vi "Smooth Move Window.vi"(8 "error in (no error)":errorcluster, 10 "Front Panel Window:Window Bounds":T1, 11 "VI in":refnum<vi>) -> (0 "error out":errorcluster, 3 "VI out":refnum<vi>)   [LabVIEW 2012, in "Win8uiDemo.lvlib" / "Flyout.lvclass"]
uses:
  Flyout.lvclass
  <vilib>/Utility/miscctls.llb/LVRectTypeDef.ctl
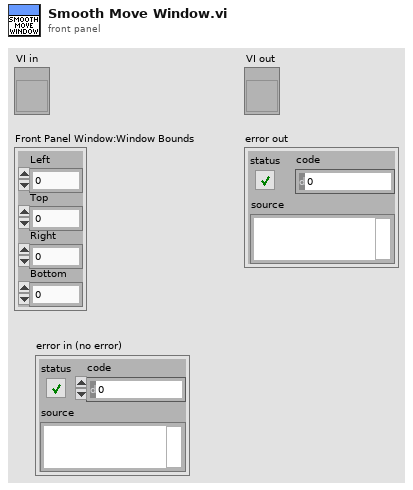
[diagram p1: front panel]
types:
  T1 = typedef "LVRectTypeDef.ctl" = cluster{"Left":i16, "Top":i16, "Right":i16, "Bottom":i16}
  T2 = cluster{"Left":dbl, "Top":dbl, "Right":dbl, "Bottom":dbl}
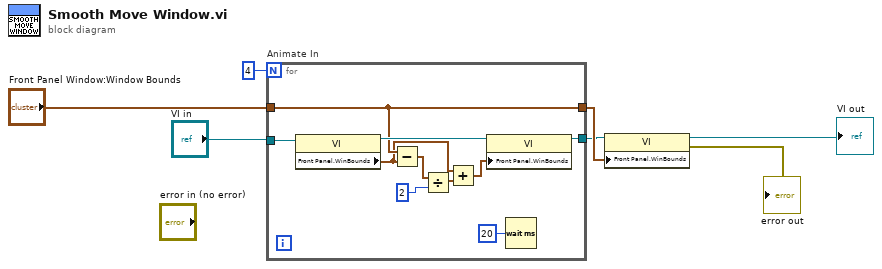
[diagram p0: block diagram]
diagram:
  n1 = for "Animate In" {
    N: 4 -> [_]
    tunnel: "VI in" -> [w17]
    tunnel: "Front Panel Window:Window Bounds" -> [w11]
    tunnel: [w12] -> w6
    tunnel: [w11] -> w7
    n2 = property class="VI"(reference=w17) -> (reference out=w13:refnum<vi>, "Front Panel.WinBounds"=w9:T1)  [unwired: 1 in, 1 out]
    n3 = Subtract(x=w11, y=w9) -> (x-y=w15:T1)
    n4 = Divide(x=w15, y=i16 2) -> (x/y=w10:T2)
    n5 = Add(x=w9, y=w10) -> (x+y=w8:T2)
    n6 = property class="VI"(reference=w13, "Front Panel.WinBounds"=w8) -> (reference out=w12:refnum<vi>)  [unwired: 1 in, 1 out]
    n7 = Wait (ms)(milliseconds to wait=u32 20) -> ()  [unwired: 1 out]
  }
  n8 = property class="VI"(reference=w6, "Front Panel.WinBounds"=w7) -> (reference out=→"VI out":refnum<vi>, error out=→"error out":errorcluster)  [unwired: 1 in]
